vi "Close Device.vi"(8 "error in (no error)":errorcluster, 11 "Thru in":refnum<class "Thru.lvclass">) -> (0 "error out":errorcluster, 3 "Thru out":refnum<class "Thru.lvclass">)   [LabVIEW 2020, in "Thru.lvclass"]
doc: "Closes the device"
uses:
  Thru.lvclass
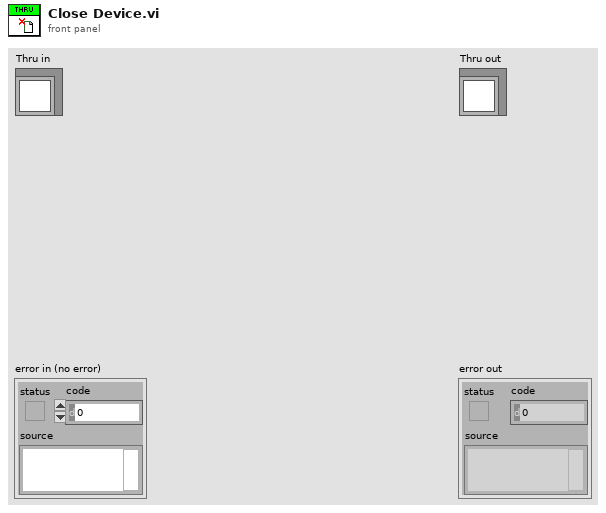
[diagram p1: front panel]
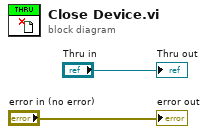
[diagram p0: block diagram]
diagram:
  "error out" <- "error in (no error)"
  "Thru out" <- "Thru in"
